vi "Update DO DAQ IO Group.vi"(7 "dCVT DAQDict":T2, 8 "error in (no error)":errorcluster, 9 "DO in":bool[](array[boolean]), 10 "DO channels":T3[](array[typedef]), 11 "DIO ClusterArray":T1[](array[typedef])) -> (0 "error out":errorcluster, 3 "DIO ClusterArray out":T1[](array[typedef]), 5 "dCVT DAQDict out":T2)   [LabVIEW 2020, in "DAQDict.lvlib"]
uses:
  DAQDict.lvlib
  support/IONameNode--cluster.ctl
  <vilib>/TELLC/Dynamic CVT API/TD Dynamic CVT DVR--ref.ctl
  support/BRS_DO - New.ctl
  support/DIO ClusterArray Element--cluster.ctl
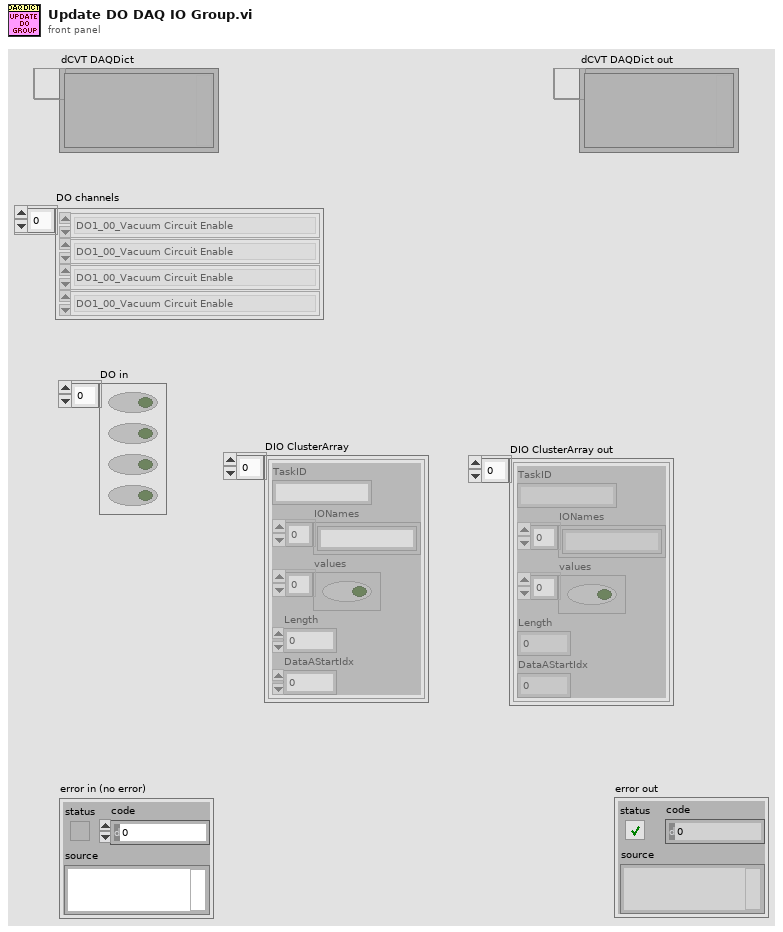
[diagram p1: front panel]
types:
  T1 = typedef "DIO ClusterArray Element--cluster.ctl" = cluster{"TaskID":string, "IONames":string[], "values":bool[], "Length":i32, "DataAStartIdx":i32}
  T2 = typedef "TD Dynamic CVT DVR--ref.ctl" = refnum<data-value>
  T3 = typedef "BRS_DO - New.ctl" = enum16{"DO1_00_Vacuum Circuit Enable", "DO1_01_Nitrogen Flow Valve Open", "DO1_02_Nitrogen Top Blow Off", "DO1_03_Nitrogen Bottom Blow Off", "DO1_04_Nitrogen Blow Off Exhaust Fan ON", "DO1_05_Signal Red Light", "DO1_06_Signal Amber Light", "DO1_07_Signal Green Light", "DO1_08_Signal Blue Light", "DO1_09_Robot Input spare 1", "DO1_10_Signal Flashing", "DO1_11_Door Interlock Solenoid Close", "DO1_12_Main Robot $CONF_MESS (Clear Error-Alarm)", "DO1_13_Main Robot $DRIVES_ON", "DO1_14_Main Robot $MOVE_ENABLE", "DO1_15_Main Robot $EXT_START (Start-Resume Program)", "DO1_16_Main Robot $DRIVES_OFF", "DO1_17_Robot Input Spare 2", "DO1_18_Robot Input Spare 3", "DO1_19_Robot Input Spare 4", "DO1_20_Robot Input Spare 5", "DO1_21_Pod Buffer Horiz Enable", "DO1_22_Pod Buffer Vert Enable", "DO1_23_Barcode Reader Backlight ON", "DO1_24_Digital Camera Image Capture", "DO1_25_BLIS ON", "DO1_26_Spare_1", "DO1_27_Spare_2", "DO1_28_Spare_3", "DO1_29_Spare_4", "DO1_30_Spare_5", "DO1_31_Spare_6", "DO2_00_Spare_7", "DO2_01_Spare_8", "DO2_02_Spare_9", "DO2_03_MLP1 Door Lock", "DO2_04_MLP1 Pod Capture", "DO2_05_MLP1 Lid Capture", "DO2_06_MLP1 Arm to Open position", "DO2_07_MLP1 Arm to Close position", "DO2_08_MLP1 Power On Indicator", "DO2_09_MLP1 Error Indicator", "DO2_10_MLP1 In Process Indicator", "DO2_11_Spare_10", "DO2_12_Spare_11", "DO2_13_Spare_12", "DO2_14_Spare_13", "DO2_15_Spare_14", "DO2_16_Spare_15", "DO2_17_Spare", "DO2_18_Spare", "DO2_19_Spare", "DO2_20_Spare", "DO2_21_Spare", "DO2_22_Spare", "DO2_23_Spare", "DO2_24_Spare", "DO2_25_Spare", "DO2_26_Spare", "DO2_27_Spare", "DO2_28_Spare", "DO2_29_Spare", "DO2_30_Spare", "DO2_31_Spare", "DO3_00_Exp1 Door Lock Solenoid Close", "DO3_01_Spare", "DO3_02_Spare", "DO3_03_Spare", "DO3_04_Spare", "DO3_05_Spare", "DO3_06_Exp1 Input Spare 1", "DO3_07_Exp1 Input Spare 2", "DO3_08_Exp1 Input Spare 3", "DO3_09_Exp1 Input Spare 4", "DO3_10_Exp1 Input Spare 5", "DO3_11_Spare", "DO3_12_Exp1 Robot $CONF_MESS (Clear Error-Alarm)", "DO3_13_Exp1 Robot $DRIVES_ON", "DO3_14_Exp1 Robot $MOVE_ENABLE", "DO3_15_Exp1 Robot $EXT_START (Start-Resume Program)", "DO3_16_Exp1 Robot $DRIVES_OFF", "DO3_17_Spare", "DO3_18_Spare", "DO3_19_Spare", "DO3_20_Spare", "DO3_21_Spare", "DO3_22_Spare", "DO3_23_Spare", "DO3_24_Spare", "DO3_25_Spare", "DO3_26_Spare", "DO3_27_Spare", "DO3_28_Spare", "DO3_29_Spare", "DO3_30_Spare", "DO3_31_Spare"}
  T4 = typedef "IONameNode--cluster.ctl" = cluster{"IOName":string, "value":bool, "IO Type":enum16{"N/A", "DI", "DO"}, "TaskID":string, "data Idx":i32}
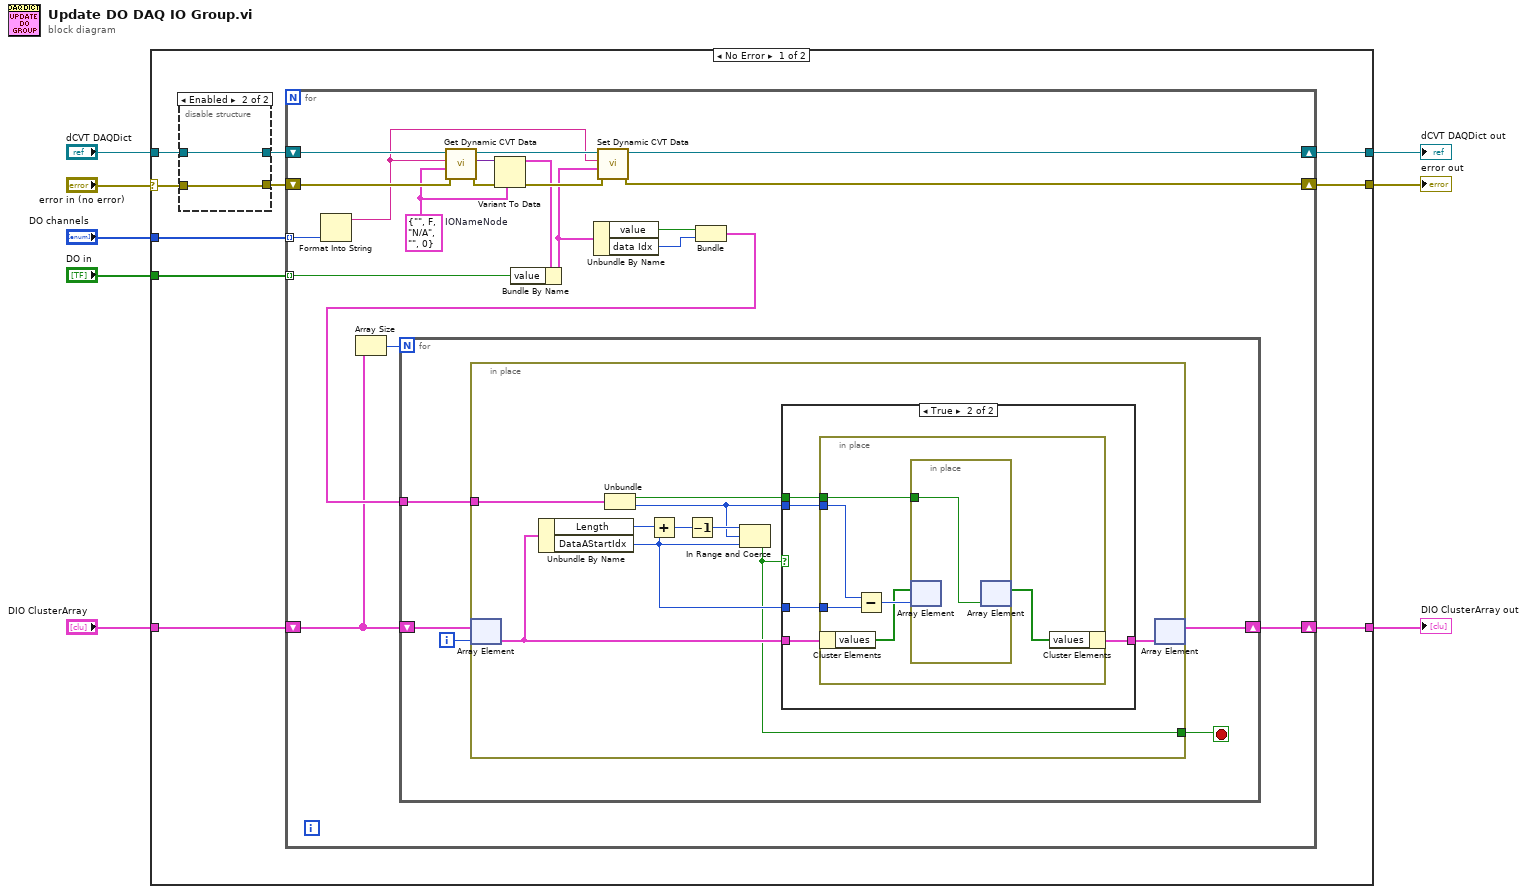
[diagram p0: block diagram]
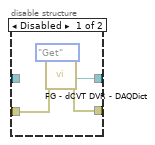
[diagram p2: hidden frame]
diagram:
  n1 = case shown="No Error" "error in (no error)" {
    selector: "error in (no error)" -> [w17 w75]
    tunnel: [w15 w75] -> w8
    tunnel: "DO channels" -> [w16 _]
    tunnel: [w14 w74] -> w5
    tunnel: "dCVT DAQDict" -> [w12 w74]
    tunnel: "DO in" -> [w11 _]
    tunnel: "DIO ClusterArray" -> [w10 w73]
    tunnel: [w9 w73] -> w2
    frame No Error {
      n2 = disable-structure shown="Enabled" {
        disable-tunnel: [w21 w23] -> w18
        disable-tunnel: w17 -> [w20 w23]
        disable-tunnel: [w19 w24] -> w13
        disable-tunnel: w12 -> [_ w24]
        frame Disabled {
          n3 = call "FG - dCVT DVR - DAQDict.vi"("error in (no error)"=w20, "Action (Get)"=enum16{"Init", "Get", "Set"}."Get") -> ("dCVT DAQDict out"=w19:T2, "error out"=w21:errorcluster)  [unwired: 7 in]
        }
        frame Enabled {
        }
      }
      n4 = for {
        shift-right: [w36] -> w14
        shift-left: w13 -> [w44]
        shift-right: [w34] -> w15
        shift-left: w18 -> [w43]
        tunnel: w16 -> [w42] mode=indexing
        tunnel: w11 -> [w30] mode=indexing
        shift-right: [w25] -> w9
        shift-left: w10 -> [w27]
        w39 = T4 {"IOName"="", "value"=FALSE, "IO Type"=enum."N/A", "TaskID"="", "data Idx"=0}  # IONameNode
        n5 = Format Into String(w42) -> (resulting string=w32:string)  [unwired: 3 in, 1 out]
        n6 = Array Size(array=w27) -> (size(s)=w26:i32)
        n7 = call <vilib>:"Get Dynamic CVT Data.vi"("error in (no error)"=w43, "default value (empty variant)"=w39, "DataName"=w32, "dCVT DVR"=w44) -> ("error out"=w40:errorcluster, "value"=w41:variant, "dCVT DVR out"=w37:T2)  [unwired: 4 in, 1 out]
        n8 = Variant To Data(error in=w40, type=w39, Variant=w41) -> (data=w33:T4, error out=w35:errorcluster)
        n9 = Bundle By Name(cluster=w33, "value"=w30) -> (w31:T4)
        n10 = Unbundle By Name(w31) -> ("value"=w38:bool, "data Idx"=w29:i32)
        n11 = call <vilib>:"Set Dynamic CVT Data.vi"("error in (no error)"=w35, "value"=w31, "DataName"=w32, "dCVT DVR"=w37) -> ("error out"=w34:errorcluster, "dCVT DVR out"=w36:T2)  [unwired: 5 in, 1 out]
        n12 = Bundle("value"=w38, "data Idx"=w29) -> (w28:cluster{"value":bool, "data Idx":i32})  [unwired: 1 in]
        n13 = for {
          N: w26 -> [_]
          tunnel: w28 -> [w49]
          shift-right: [w47] -> w25
          shift-left: w27 -> [w48]
          i -> [w46]
          stop <- w45 stop-if-true
          n14 = in-place {
            in-place-border: w49 -> [w56]
            in-place-border: [w51] -> w45
            n15 = in-place-array #1(w48, w46) -> (w52:T1)
            n16 = Unbundle By Name(w52) -> ("Length"=w58:i32, "DataAStartIdx"=w53:i32)
            n17 = Unbundle(w56) -> ("value"=w55:bool, "data Idx"=w54:i32)
            n18 = Add(x=w58, y=w53) -> (x+y=w59:i32)
            n19 = Decrement(x=w59) -> (x-1=w57:i32)
            n20 = In Range and Coerce(upper limit=w57, x=w54, lower limit=w53) -> (In Range?=w51:bool)  [unwired: 1 out]
            n21 = case shown="True" w51 {
              tunnel: w55 -> [_ w64]
              tunnel: w54 -> [_ w63]
              tunnel: w52 -> [w60 w65]
              tunnel: w53 -> [_ w62]
              tunnel: [w60 w61] -> w50
              frame False {
              }
              frame True {
                n22 = in-place {
                  in-place-border: w64 -> [w67]
                  in-place-border: w63 -> [w69]
                  in-place-border: w62 -> [w70]
                  n23 = in-place-cluster #2(w65) -> ("values"=w68:bool[])
                  n24 = Subtract(x=w69, y=w70) -> (x-y=w71:i32)
                  n25 = in-place {
                    in-place-border: w67 -> [w72]
                    n26 = in-place-array #3(w68, w71) -> ()  [unwired: 1 out]
                    n27 = in-place-array #3(w72) -> (w66:bool[])  [unwired: 1 out]
                  }
                  n28 = in-place-cluster #2("values"=w66) -> (w61:T1)
                }
              }
            }
            n29 = in-place-array #1(w50) -> (w47:T1[])  [unwired: 1 out]
          }
        }
      }
    }
    frame Error {
    }
  }
  "error out" <- w8
  "dCVT DAQDict out" <- w5
  "DIO ClusterArray out" <- w2
